vi "Parse Message.vi"(1 "Listener Message":T2={"Listener Command"=enum."Close", "Value"=variant}) -> (5 "Listener Command":T1=enum."Open", 7 "Value":variant)   [LabVIEW 2019, in "Listener.lvlib"]
uses:
  Listener.lvlib
  Listener Message.ctl
  Listener Command.ctl
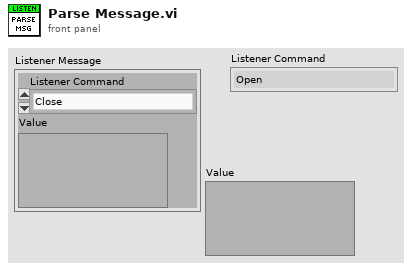
[diagram p1: front panel]
types:
  T1 = typedef "Listener.lvlib/Listener Command.ctl" = enum16{"Idle", "Open", "Incoming", "Close", "Error", "Stop"}
  T2 = typedef "Listener.lvlib/Listener Message.ctl" = cluster{"Listener Command":T1, "Value":variant}
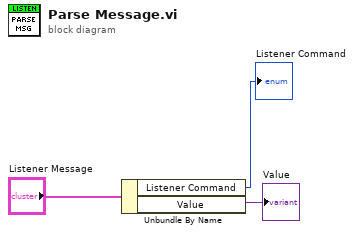
[diagram p0: block diagram]
diagram:
  n1 = Unbundle By Name("Listener Message") -> ("Listener Command"=→"Listener Command":T1, "Value"=→"Value":variant)
